vi "Get Info.vi"(8 "error in (no error)":errorcluster, 11 "Hardware in":refnum<class "Hardware.lvclass">) -> (0 "error out":errorcluster, 2 "Info":variant, 3 "Hardware out":refnum<class "Hardware.lvclass">)   [LabVIEW 2020, in "Instrument.lvlib" / "Hardware.lvclass"]
uses:
  Hardware.lvclass
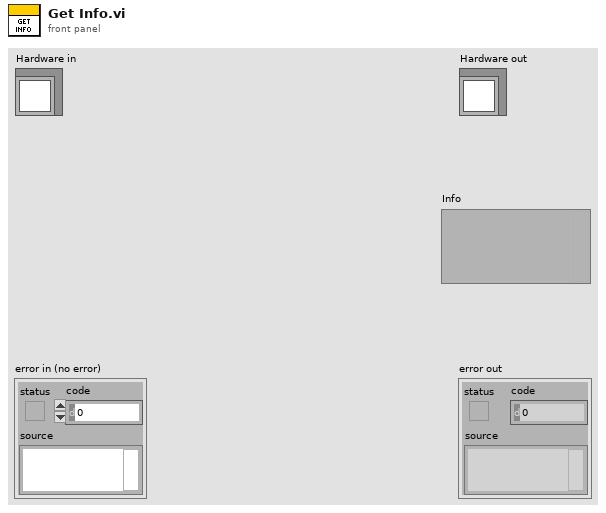
[diagram p1: front panel]
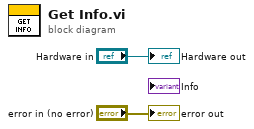
[diagram p0: block diagram]
diagram:
  "error out" <- "error in (no error)"
  "Hardware out" <- "Hardware in"
